vi "Inline Write (Objects).vi"(8 "error in":errorcluster, 11 "RT State Variables in":T1 {"runtime data"."out object status BD"."Data Reference" format="%.0x"; "runtime data"."out object data BD"."Data Reference" format="%.0x"; "runtime data"."out interaction status BD"."Data Reference" format="%.0x"; "runtime data"."out interaction data BD"."Data Reference" format="%.0x"; "Settings"."objectData"."out object status BD"."Data Reference" format="%.0x"; "Settings"."objectData"."out object data BD"."Data Reference" format="%.0x"; "Settings"."objectData"."out interaction status BD"."Data Reference" format="%.0x"; "Settings"."objectData"."out interaction data BD"."Data Reference" format="%.0x"}) -> (0 "error out":errorcluster, 3 "RT State Variables out":T1 {"runtime data"."out object status BD"."Data Reference" format="%.0x"; "runtime data"."out object data BD"."Data Reference" format="%.0x"; "runtime data"."out interaction status BD"."Data Reference" format="%.0x"; "runtime data"."out interaction data BD"."Data Reference" format="%.0x"; "Settings"."objectData"."out object status BD"."Data Reference" format="%.0x"; "Settings"."objectData"."out object data BD"."Data Reference" format="%.0x"; "Settings"."objectData"."out interaction status BD"."Data Reference" format="%.0x"; "Settings"."objectData"."out interaction data BD"."Data Reference" format="%.0x"})   [LabVIEW 2019, in "HLA Custom Device Engine.lvlib"]
uses:
  HLA Custom Device Engine.lvlib
  RTStateVariables.ctl
  <vilib>/NI/NIVS Inline Async API/_VS Inline Async API/VS Inline Async API/VS Inline Async API.lvclass
  Shared/Compiled.Settings.ctl
  Shared/main_page_config.ctl
  Shared/object_managament_config.ctl
  Shared/interaction_parameter_configuration.ctl
  Shared/object_attribute_configuration.ctl
  Shared/object_status_info.ctl
  Shared/object_data.ctl
  <vilib>/NI VeriStand/Custom Device API/Block Data Reference.ctl
  <vilib>/NI VeriStand/Custom Device API/Data Reference.ctl
  RTruntimeData.ctl
  _typedefs/RThlaMapHelpers.ctl
  _typedefs/map_in_interaction.ctl
  _typedefs/map_interaction_value.ctl
  _typedefs/map_attr_param_data.ctl
  _typedefs/map_object.ctl
  _typedefs/map_object_key.ctl
  _typedefs/map_object_value.ctl
  _typedefs/map_object_instance.ctl
  _typedefs/map_object_instance_value.ctl
  _typedefs/map_object_vs_instance.ctl
  _typedefs/map_out_vs_ch_instanceId.ctl
  _typedefs/map_out_vs_ch_objects.ctl
  _typedefs/map_out_vs_ch_objects_value.ctl
  _typedefs/map_out_vs_ch_interactIonClass.ctl
  emea-ni-adg-hla-lv/src/library/typedefs/receiveInteractionEvent_type.ctl
  emea-ni-adg-hla-lv/src/library/typedefs/OrderType.ctl
  emea-ni-adg-hla-lv/src/library/typedefs/TransportationType.ctl
  emea-ni-adg-hla-lv/src/library/typedefs/reflectAttributeValuesEvent_type.ctl
  emea-ni-adg-hla-lv/src/library/typedefs/discoverObjectInstanceEvent_type.ctl
  emea-ni-adg-hla-lv/src/library/typedefs/removeObjectInstanceEvent_type.ctl
  <vilib>/NI VeriStand/Custom Device API/Global Data Refs.vi
  <vilib>/NI VeriStand/Custom Device API/Custom Device API.lvlib
  Data Encoding_Decoding/HLA Data Conversion.lvlib
  _Debug/VsDebugLibrary.lvlib
  emea-ni-adg-hla-lv/src/library/openrti_rti1516eLv.lvlib
  emea-ni-adg-hla-lv/src/helpers/Attribute Handle Value Map/ahvm.lvlib
  Shared/HLA Custom Device Shared.lvlib
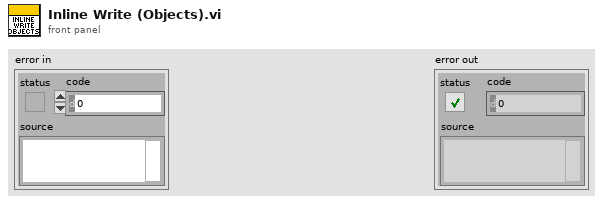
[diagram p1: front panel]
types:
  T1 = typedef "HLA Custom Device Engine.lvlib/RTStateVariables.ctl" = cluster{"Async":refnum<class "VS Inline Async API.lvclass">, "Settings":T2, "runtime data":T11}
  T2 = typedef "HLA Custom Device Shared.lvlib/Compiled.Settings.ctl" = cluster{"Name":string, "Async Init Timeout":u16, "main page properties":T3, "obiectConfig":T4, "objectStatus":T7, "objectData":T8}
  T3 = typedef "HLA Custom Device Shared.lvlib/main_page_config.ctl" = cluster{"Federate Execution Name":string, "Federate Type":string, "Local Designator Settings":string, "FOM Module":path, "mak mtl file":path, "FOM destination path":string}
  T4 = typedef "HLA Custom Device Shared.lvlib/object_managament_config.ctl" = cluster{"incoming interactions":T5[], "incoming objects":T6[], "outgoing interactions":T5[], "outgoing objects":T6[]}
  T5 = typedef "HLA Custom Device Shared.lvlib/interaction_parameter_configuration.ctl" = cluster{"interaction class name":string, "parameter name":string, "datatype":string, "vsChIndex":i32, "vsChName":string}
  T6 = typedef "HLA Custom Device Shared.lvlib/object_attribute_configuration.ctl" = cluster{"object class name":string, "instanceId":i32, "attribute name":string, "datatype":string, "vsChIndex":i32, "vsChName":string}
  T7 = typedef "HLA Custom Device Shared.lvlib/object_status_info.ctl" = cluster{"incoming interactions":map{string, map{string, i32}}, "incoming objects":map{string, map{string, i32}}, "outgoing interactions":map{string, map{string, i32}}, "outgoing objects":map{string, map{string, i32}}}
  T8 = typedef "HLA Custom Device Shared.lvlib/object_data.ctl" = cluster{"out interaction data BD":T9[], "out interaction data size":i32, "out interaction status BD":T9[], "out interaction status size":i32, "out object data BD":T9[], "out object data size":i32, "out object status BD":T9[], "out object status size":i32}
  T9 = typedef "Custom Device API.lvlib/Block Data Reference.ctl" = cluster{"Data Reference":T10, "Offset":u64, "Length":u64}
  T10 = typedef "Custom Device API.lvlib/Data Reference.ctl" = i32
  T11 = typedef "HLA Custom Device Engine.lvlib/RTruntimeData.ctl" = cluster{"rtiHandle":i64, "hlaMap":T12, "hla event registration":refnum<event-registration>, "out interaction data BD":T9[], "out interaction data":dbl[], "out interaction status BD":T9[], "out interaction status ":dbl[], "out object data BD":T9[], "out object data":dbl[], "out object status BD":T9[], "out object status ":dbl[]}
  T12 = typedef "HLA Custom Device Engine.lvlib/RThlaMapHelpers.ctl" = cluster{"in_interactionMap":T13, "in_objectMap":T16, "in_map_object_instance":T19, "in_map_vs_incoming_instance":T21, "out_map_vs_ch_instanceId":T22, "out_interactionMap":T13, "out_map_vs_ch_objectInstance":T23, "out_objectMap":T16, "out_map_vs_ch_interactionClass":T25}
  T13 = typedef "HLA Custom Device Engine.lvlib/map_in_interaction.ctl" = map{u64, T14}
  T14 = typedef "HLA Custom Device Engine.lvlib/map_interaction_value.ctl" = cluster{"infoChMap":map{string, i32}, "parameterMap":map{u64, T15}, "parHandleValueMap":u64}
  T15 = typedef "HLA Custom Device Engine.lvlib/map_attr_param_data.ctl" = cluster{"dataType":string, "index":i32}
  T16 = typedef "HLA Custom Device Engine.lvlib/map_object.ctl" = map{T17, T18}
  T17 = typedef "HLA Custom Device Engine.lvlib/map_object_key.ctl" = cluster{"instanceId":i32, "objectClassHandle":u64}
  T18 = typedef "HLA Custom Device Engine.lvlib/map_object_value.ctl" = cluster{"infoChMap":map{string, i32}, "attributeMap":map{u64, T15}, "attrHandleSet":u64, "attrHandleValueMap":u64, "objectInstancePrefix":string}
  T19 = typedef "HLA Custom Device Engine.lvlib/map_object_instance.ctl" = map{u64, T20}
  T20 = typedef "HLA Custom Device Engine.lvlib/map_object_instance_value.ctl" = cluster{"objectClassHandle":u64, "objectInstanceName":string, "InstanceID":i32}
  T21 = typedef "HLA Custom Device Engine.lvlib/map_object_vs_instance.ctl" = map{u64, map{i32, u64}}
  T22 = typedef "HLA Custom Device Engine.lvlib/map_out_vs_ch_instanceId.ctl" = map{i32, i32}
  T23 = typedef "HLA Custom Device Engine.lvlib/map_out_vs_ch_objects.ctl" = map{i32, T24}
  T24 = typedef "HLA Custom Device Engine.lvlib/map_out_vs_ch_objects_value.ctl" = cluster{"ObjectInstance":u64, "ObjectClass":u64}
  T25 = typedef "HLA Custom Device Engine.lvlib/map_out_vs_ch_interactIonClass.ctl" = map{i32, u64}
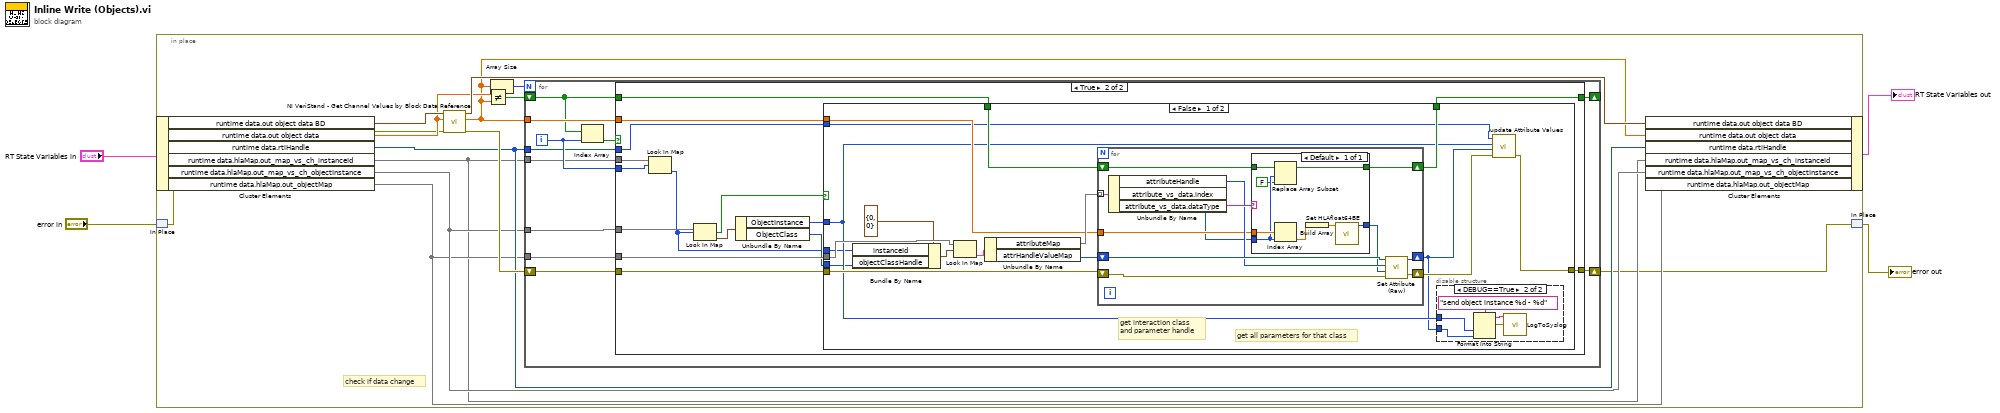
[diagram p0: block diagram]
diagram:
  n1 = in-place {
    # "check if data change"
    n2 = in-place-cluster #1("RT State Variables in") -> ("runtime data.out object data BD"=w17:T9[], "runtime data.out object data"=w9:dbl[], "runtime data.rtiHandle"=w12:i64, "runtime data.hlaMap.out_map_vs_ch_instanceId"=w7:T22, "runtime data.hlaMap.out_map_vs_ch_objectInstance"=w11:T23, "runtime data.hlaMap.out_objectMap"=w10:T16)
    n3 = in-place-match #2("error in") -> (w6:errorcluster)
    n4 = call <vilib>:"NI VeriStand - Get Channel Values by Block Data Reference.vi"("error in (no error)"=w6, "Values Array in"=w9, "Block Data Ref"=w17) -> ("error out"=w15:errorcluster, "Values Array out"=w8:dbl[], "Block Data Ref dup"=w16:T9[])  [unwired: 6 in]
    n5 = Not Equal?(x=w9, y=w8) -> (x != y?=w14:bool[])
    n6 = Array Size(array=w8) -> (size(s)=w13:i32)
    n7 = for {
      N: w13 -> [_]
      tunnel: w11 -> [w27]
      tunnel: w10 -> [w26]
      tunnel: w8 -> [w24]
      shift-right: [w28] -> w5
      shift-left: w15 -> [w25]
      shift-right: [w20] -> _
      shift-left: w14 -> [w23]
      tunnel: w12 -> [w19]
      tunnel: w7 -> [w18]
      i -> [w21]
      n8 = Index Array(array=w23, index=w21) -> (element=w22:bool)
      n9 = case shown="True" w22 {
        tunnel: [w30 w39] -> w28
        tunnel: w27 -> [_ w45]
        tunnel: w26 -> [_ w44]
        tunnel: w25 -> [w30 w43]
        tunnel: w24 -> [_ w42]
        tunnel: w23 -> [w29 w41]
        tunnel: w21 -> [_ w32]
        tunnel: [w29 w40] -> w20
        tunnel: w19 -> [_ w38]
        tunnel: w18 -> [_ w33]
        frame False {
        }
        frame True {
          n10 = Look In Map(map=w33, key=w32) -> (value=w31:i32)  [unwired: 1 in, 1 out]
          n11 = Look In Map(map=w45, key=w31) -> (key not found?=w36:bool, value=w37:T24)  [unwired: 1 in]
          n12 = Unbundle By Name(w37) -> ("ObjectInstance"=w34:u64, "ObjectClass"=w35:u64)
          n13 = case shown="False" w36 {
            tunnel: w44 -> [w62 _]
            tunnel: w43 -> [w58 w88]
            tunnel: w42 -> [w57 _]
            tunnel: w41 -> [w56 w89]
            tunnel: [w55 w89] -> w40
            tunnel: [w53 w88] -> w39
            tunnel: w38 -> [w52 _]
            tunnel: w35 -> [w48 _]
            tunnel: w34 -> [w51 _]
            tunnel: w31 -> [w47 _]
            frame False {
              # "get all parameters for that class"
              # "get interaction class\nand parameter handle"
              n14 = Bundle By Name(cluster=T17 {"instanceId"=0, "objectClassHandle"=0} ("key"), "instanceId"=w47, "objectClassHandle"=w48) -> (w49:T17)
              n15 = Look In Map(map=w62, key=w49) -> (value=w61:T18)  [unwired: 1 in, 1 out]
              n16 = Unbundle By Name(w61) -> ("attributeMap"=w59:map{u64, T15}, "attrHandleValueMap"=w60:u64)
              n17 = for {
                shift-right: [w73] -> w46
                shift-left: w60 -> [w78]
                tunnel: w59 -> [w79] mode=indexing
                shift-right: [w75] -> w54
                shift-left: w58 -> [w77]
                tunnel: w57 -> [w72]
                shift-right: [w68] -> w55
                shift-left: w56 -> [w69]
                n18 = Unbundle By Name(w79) -> ("attributeHandle"=w74:u64, "attribute_vs_data.index"=w71:i32, "attribute_vs_data.dataType"=w76:string)
                n19 = case shown="Default" w76 {
                  tunnel: w72 -> [w87]
                  tunnel: w71 -> [w82]
                  tunnel: [w84] -> w70
                  tunnel: w69 -> [w83]
                  tunnel: [w80] -> w68
                  frame Default {
                    n20 = Replace Array Subset(array=w83, new element=FALSE ("new element/subarray"), index=w82) -> (w80:bool[])
                    n21 = Index Array(array=w87, index=w82) -> (element=w86:dbl)
                    n22 = Build Array(w86) -> (w85:dbl[])
                    n23 = call "Set HLAfloat64BE.vi"("eu data in"=w85) -> ("raw data out"=w84:u8[])  [unwired: 9 in, 1 out]
                  }
                }
                n24 = call "Set Attribute (Raw).vi"("error in"=w77, "data"=w70, "attributeHandle in"=w74, "attrHandleValueMap in"=w78) -> ("error out"=w75:errorcluster, "attrHandleValueMap out"=w73:u64)  [unwired: 5 in, 1 out]
              }
              n25 = disable-structure shown="DEBUG==True" {
                disable-tunnel: w51 -> [_ w64]
                disable-tunnel: w46 -> [_ w63]
                frame condition #0 {
                }
                frame condition #1 (active) {
                  n26 = Format Into String(format string="send object instance %d - %d", w64, w63) -> (resulting string=w66:string, error out=w67:errorcluster)  [unwired: 2 in]
                  n27 = call "LogToSyslog.vi"("error in (no error)"=w67, "message"=w66) -> ()  [unwired: 8 in, 2 out]
                }
              }
              n28 = call "update Attribute Values.vi"("error in"=w54, "attributeHandleValueMap in"=w46, "objectInstanceHandle in"=w51, "rtiHandle in"=w52) -> ("error out"=w53:errorcluster)  [unwired: 4 in, 3 out]
            }
            frame True {
            }
          }
        }
      }
    }
    n29 = in-place-cluster #1("runtime data.out object data BD"=w16, "runtime data.out object data"=w8, "runtime data.rtiHandle"=w12, "runtime data.hlaMap.out_map_vs_ch_instanceId"=w7, "runtime data.hlaMap.out_map_vs_ch_objectInstance"=w11, "runtime data.hlaMap.out_objectMap"=w10) -> (→"RT State Variables out":T1)
    n30 = in-place-match #2(w5) -> (→"error out":errorcluster)
  }
